vi "Nested Malleable VIs - Lesson 2b.vi"() -> ()   [LabVIEW 2023]
doc: "Lesson 2b continues Lesson 2 with one further example of the flexibility offered by malleable VIs when working with complex data types."
uses:
  String With Equals/String With Equals.lvclass/String With Equals.ctl
  String Without Equals/String Without Equals.lvclass/String Without Equals.ctl
  763d4b9c-944e-4acb-82a1-ce50c1d65406.vi
  fd91f596-61ba-4296-af35-812e4d4f2264.vi
  fd91f596-61ba-4296-af35-812e4d4f2264.vi/529e3ff3-7b1a-4637-8f9b-fb3c31bc4e4f.vi
  fd91f596-61ba-4296-af35-812e4d4f2264.vi/529e3ff3-7b1a-4637-8f9b-fb3c31bc4e4f.vi/5d3ee391-5e24-46f3-8538-f76ba2ee4917.vi
  String With Equals/Equals.vi
  String With Equals/String With Equals.lvclass
  String Without Equals/String Without Equals.lvclass
  <vilib>/Comparison/Equal/Equal Functor/Equal Functor.lvclass
panel:
  out "index of element 2":i32
  out "index of element 1":i32
  # "Overview: This VI simply continues Lesson 2 with one further example of the possible flexibility of malleable VIs when working with complex data types.\n\nInstructions: \n1. Open the block diagram of this VI. Review the lessons presented there.\n2. Run the VI to see the results. \n3. Once you have finished reviewing this VI, open the next lesson VI in the Malleable VIs - Nested Malleable VIs example project."
  # "This one finds the element at index 1."
  # "This one does not find the element and so returns -1."
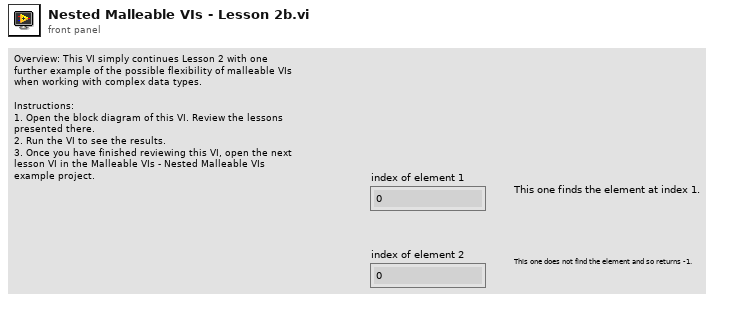
[diagram p1: front panel]
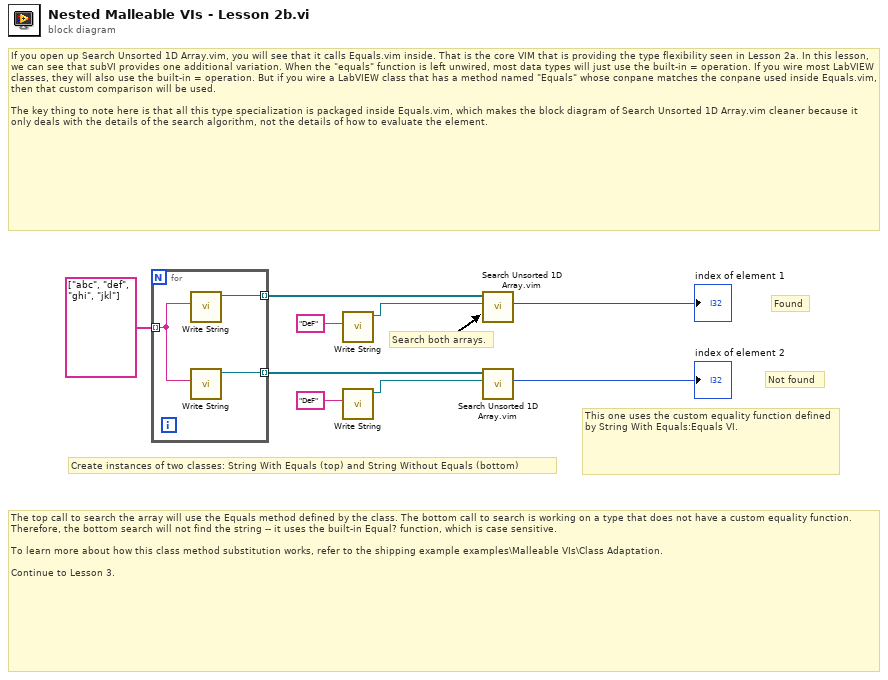
[diagram p0: block diagram]
diagram:
  # "Found"
  # "Not found"
  # "The top call to search the array will use the Equals method defined by the class. The bottom call to search is working on a type that does not have a custom equality function. Therefore, the bottom search will not find the string -- it uses the built-in Equal? function, which is case sensitive.\n\nTo learn more about how this class method substitution works, refer to the shipping example examples\\Malleable VIs\\Class Adaptation.\n\nContinue to Lesson 3."
  # "This one uses the custom equality function defined by String With Equals:Equals VI."
  # "Search both arrays."
  # "Create instances of two classes: String With Equals (top) and String Without Equals (bottom)"
  # "If you open up Search Unsorted 1D Array.vim, you will see that it calls Equals.vim inside. That is the core VIM that is providing the type flexibility seen in Lesson 2a. In this lesson, we can see that subVI provides one additional variation. When the \"equals\" function is left unwired, most data types will just use the built-in = operation. If you wire most LabVIEW classes, they will also use the built-in = operation. But if you wire a LabVIEW class that has a method named \"Equals\" whose conpane matches the conpane used inside Equals.vim, then that custom comparison will be used. \n\nThe key thing to note here is that all this type specialization is packaged inside Equals.vim, which makes the block diagram of Search Unsorted 1D Array.vim cleaner because it only deals with the details of the search algorithm, not the details of how to evaluate the element."
  n1 = for {
    tunnel: string[] ["abc", "def", "ghi", "jkl"] ("1D array") -> [w12] mode=indexing
    tunnel: [w11] -> w7 mode=indexing
    tunnel: [w10] -> w1 mode=indexing
    n2 = call "Write String.vi"("string"=w12) -> ("String With Equals"=w11:refnum<class "String With Equals.lvclass">)  [unwired: 10 in]
    n3 = call "Write String.vi"("string"=w12) -> ("String Without Equals"=w10:refnum<class "String Without Equals.lvclass">)  [unwired: 10 in]
  }
  n4 = call "Write String.vi"("string"="DeF") -> ("String With Equals"=w5:refnum<class "String With Equals.lvclass">)  [unwired: 10 in]
  n5 = call "Write String.vi"("string"="DeF") -> ("String Without Equals"=w4:refnum<class "String Without Equals.lvclass">)  [unwired: 10 in]
  n6 = call "Search Unsorted 1D Array.vim"("element"=w5, "unsorted 1D array"=w7) -> ("index of element"=→"index of element 1":i32)  [unwired: 9 in]
  n7 = call "Search Unsorted 1D Array.vim"("element"=w4, "unsorted 1D array"=w1) -> ("index of element"=→"index of element 2":i32)  [unwired: 9 in]
